vi "PowerOverTime.vi"() -> ()   [LabVIEW 2009]
uses:
  <vilib>/Utility/file.llb/Write To Spreadsheet File (DBL).vi
panel:
  out "Current Time (Hours)":dbl
  out "Current Chart":dbl(graph)
  out "Voltage Chart":T1(graph)
  out "Power Chart":dbl(graph)
  out "Power":dbl
  out "Current":dbl
  out "Voltage":dbl
  out "Numeric":i32
  in  "stop":bool
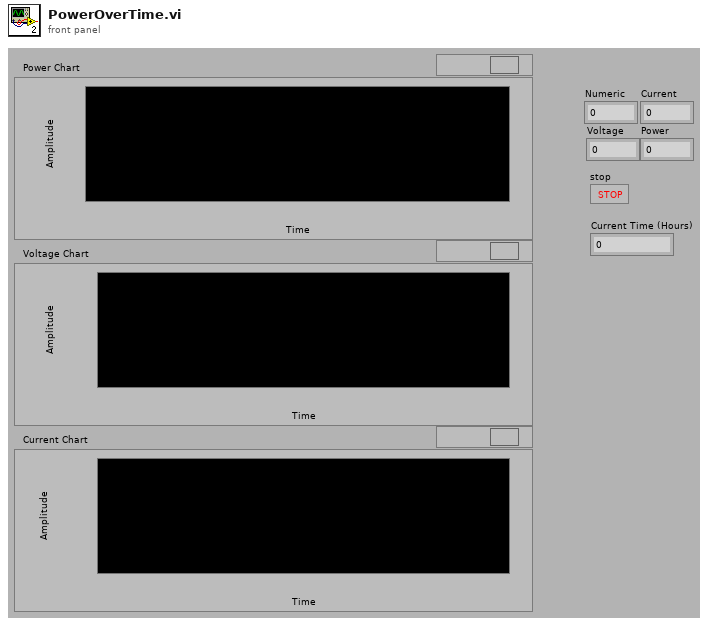
[diagram p1: front panel]
types:
  T1 = cluster{"Voltage":dbl, "Current":dbl, "Power":dbl, "WattHours":dbl}
  T2 = cluster{"Voltage":dbl, "Current":dbl, "Power":dbl, "WattHours":dbl}[]
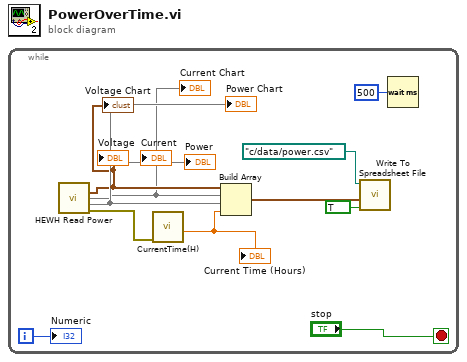
[diagram p0: block diagram]
diagram:
  n1 = while {
    i -> [w8]
    stop <- "stop" stop-if-true
    n2 = call "HEWH Read Power.vi"() -> ("PowerData"=w5:T1, 8:w4, 10:w6, "error out"=w2:errorcluster)  [unwired: 10 in, 2 out]
    "Voltage" <- w5
    "Current" <- w4
    "Power" <- w6
    "Power Chart" <- w6
    "Voltage Chart" <- w5
    "Current Chart" <- w4
    n3 = call "CurrentTime(H).vi"("error in (no error)"=w2) -> ("Current Time (Hours)"=w3:dbl)  [unwired: 9 in, 1 out]
    "Current Time (Hours)" <- w3
    n4 = Build Array(w5, w4, w6, w3) -> (w7:T2)
    n5 = call-poly <vilib>:"Write To Spreadsheet File.vi"("append to file? (new file:F)"=TRUE, "1D data"=w7, "file path (dialog if empty)"=path "c:/data/power.csv") -> ()  [unwired: 5 in, 1 out]
    n6 = Wait (ms)(milliseconds to wait=u32 500) -> ()  [unwired: 1 out]
    "Numeric" <- w8
  }
